vi "Coord window-Bring to front and list focus.vi"   [LabVIEW 2017]
uses:
  Globals/Coord window-Globals.vi
types:
  T1 = enum32{"Invalid", "Standard", "Closed", "Hidden", "Minimized", "Maximized"}
  T2 = typedef "Coordinate list window refs.ctl" = cluster{"Window Name (i.e. Key)":string, "menu reference":refnum<k9>, "VI's reference":refnum<vi>, "Pane 1":refnum<vi>, "Pane 2":refnum<vi>, "Coord Listbox":refnum<vi>, "File name":refnum<vi>, "Picture Map":refnum<vi>, "Stage XYZ Position ind.":refnum<vi>}
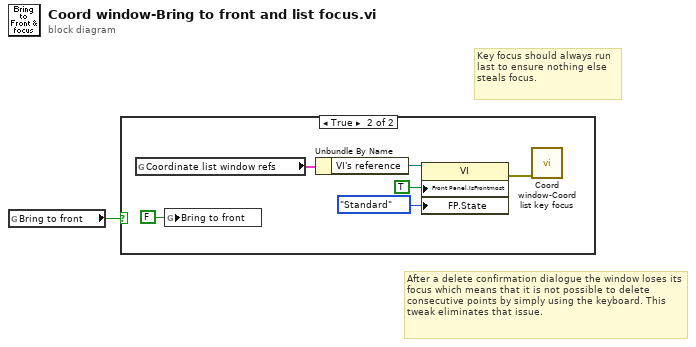
[diagram p0: block diagram]
diagram:
  # "After a delete confirmation dialogue the window loses its focus which means that it is not possible to delete consecutive points by simply using the keyboard. This tweak eliminates that issue."
  # "Key focus should always run last to ensure nothing else steals focus."
  n1 = global read "Coord window-Globals.vi" "Bring to front"() -> (w1:bool)
  n2 = case shown="True" w1 {
    frame False {
    }
    frame True {
      n3 = global read "Coord window-Globals.vi" "Coordinate list window refs"() -> (w2:T2)
      n4 = global write "Coord window-Globals.vi" "Bring to front"(FALSE ("Bring to front")) -> ()
      n5 = Unbundle By Name(w2) -> ("VI's reference"=w3:refnum<vi>)
      n6 = property class="VI"(reference=w3, "Front Panel.IsFrontmost"=TRUE ("Front Panel Window:Is Frontmost"), "FP.State"=T1."Standard" ("Front Panel Window:State")) -> (error out=w4:errorcluster)  [unwired: 1 in, 1 out]
      n7 = call "Coord window-Coord list key focus.vi"("error in (no error)"=w4) -> ()  [unwired: 10 in, 1 out]
    }
  }
